vi "TwoEdge (subVI).vi"(1 "Input 1":bool, 2 "Input 0":bool) -> (0 "Edge Separation (ms)":u32)   [LabVIEW 2015]
doc: "This subVI supports a two-edge counter application. It finds the difference between rising edges of Input 0 and Input 1 and reports in milliseconds. It also indicates when the input edges are detected by illuminating the corresponding LED on the evaluation board (LED 0 for an edge on Input 0 and LED 1 after an edge on Input 1)."
panel:
  # "This subVI supports a two-edge counter application.  It finds the difference between rising edges of Input 0 and Input 1 and reports in milliseconds.  It also indicates when the input edges are detected by illuminating the corresponding LED on the evaluation board (LED 0 for an edge on Input 0 and LED 1 after an edge on Input 1)."
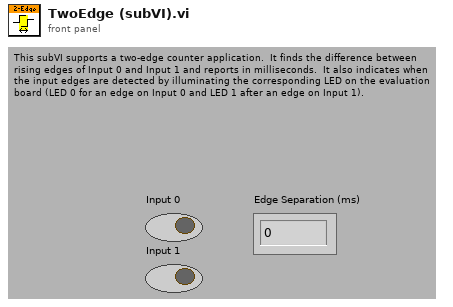
[diagram p1: front panel]
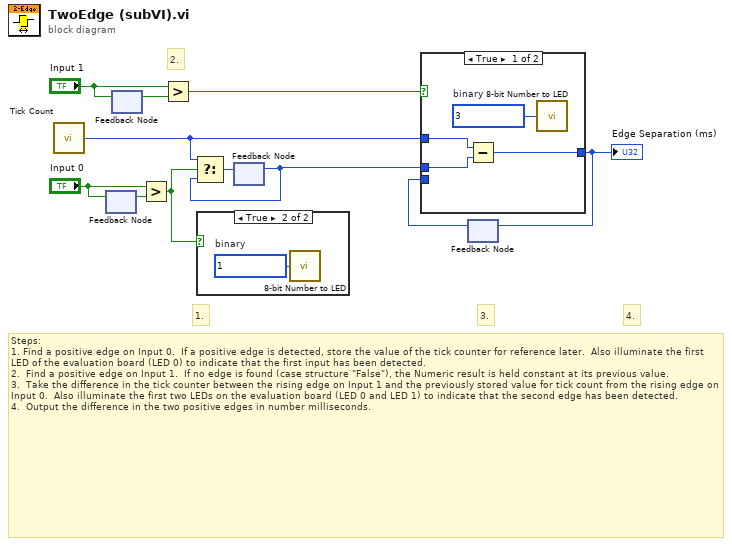
[diagram p0: block diagram]
diagram:
  # "4."
  # "3."
  # "2."
  # "1."
  # "Steps:\n1. Find a positive edge on Input 0.  If a positive edge is detected, store the value of the tick counter for reference later.  Also illuminate the first LED of the evaluation board (LED 0) to indicate that the first input has been detected. \n2.  Find a positive edge on Input 1.  If no edge is found (case structure \"False\"), the Numeric result is held constant at its previous value.\n3.  Take the difference in the tick counter between the rising edge on Input 1 and the previously stored value for tick count from the rising edge on Input 0.  Also illuminate the first two LEDs on the evaluation board (LED 0 and LED 1) to indicate that the second edge has been detected.\n4.  Output the difference in the two positive edges in number milliseconds."
  n1 = call "Tick Count"() -> ("Tick Count(mSec)"=w11:u32)
  n2 = feedback-in #1("Input 0") -> ()
  n3 = feedback #1() -> (w8:bool)  [unwired: 1 out]
  n4 = feedback-in #2("Input 1") -> ()
  n5 = feedback #2() -> (w7:bool)  [unwired: 1 out]
  n6 = Greater?(x="Input 0", y=w8) -> (0:w1:bool)
  n7 = Greater?(x="Input 1", y=w7) -> (0:w10:bool)
  n8 = case shown="True" w1 {
    frame False {
    }
    frame True {
      w12 = u8 1  # binary
      n9 = call "8-bit Number to LED.vi"("6-bit Unsigned\n Number (0-63)"=w12) -> ()  [unwired: 1 out]
    }
  }
  n10 = feedback #3() -> (w2:u32)  [unwired: 1 out]
  n11 = Select(t=w11, s=w1, f=w2) -> (s? t:f=w3:u32)
  n12 = feedback-in #3(w3) -> ()
  n13 = feedback #4() -> (w4:u32)  [unwired: 1 out]
  n14 = case shown="True" w10 {
    tunnel: w4 -> [_ w17]
    tunnel: w11 -> [w15 _]
    tunnel: [w16 w17] -> w5
    tunnel: w2 -> [w14 _]
    frame True {
      w13 = u8 3  # binary
      n15 = Subtract(x=w15, y=w14) -> (x-y=w16:u32)
      n16 = call "8-bit Number to LED.vi"("6-bit Unsigned\n Number (0-63)"=w13) -> ()  [unwired: 1 out]
    }
    frame False {
    }
  }
  "Edge Separation (ms)" <- w5
  n17 = feedback-in #4(w5) -> ()
